vi "Destroy.vi"(8 "error in (no error)":errorcluster caption="错误输入（无错误）", 11 "User Event Collection 输入":refnum<class "User Event Collection.lvclass"> caption="DNL_LabVIEW Object in") -> (0 "error out":errorcluster caption="错误输出", 3 "User Event Collection 输出":refnum<class "User Event Collection.lvclass"> caption="DNL_LabVIEW Object out")   [LabVIEW 2013, in "User Event Collection.lvclass"]
uses:
  User Event Collection.lvclass
  User Event Collection.lvclass/User Event Collection.ctl
  <resource>/importtools/Common/Event/NISAST Event.lvclass
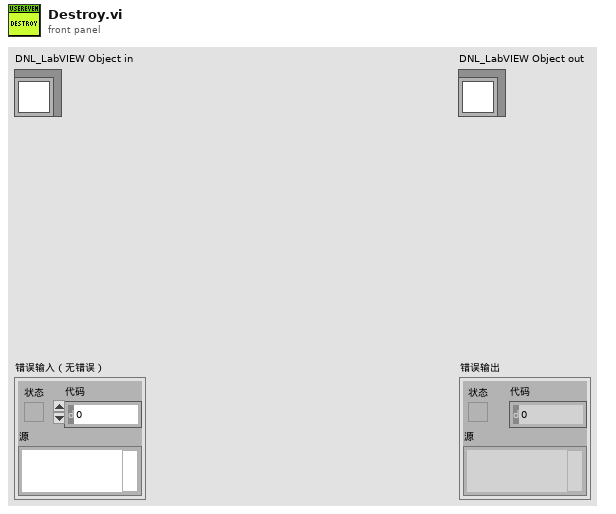
[diagram p1: front panel]
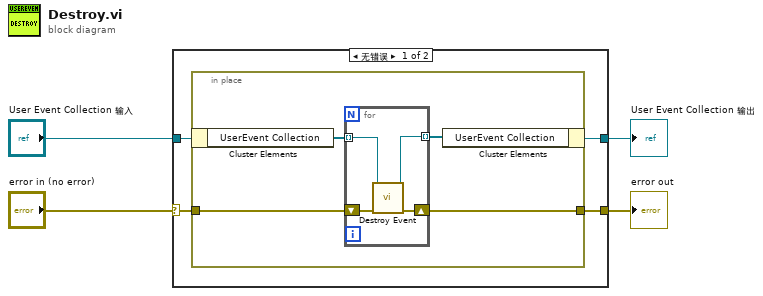
[diagram p0: block diagram]
diagram:
  n1 = case shown="无错误" "error in (no error)" {
    selector: "error in (no error)" -> [w8 w18]
    tunnel: [w7 w18] -> w3
    tunnel: [w5 w17] -> w1
    tunnel: "User Event Collection 输入" -> [w6 w17]
    frame No Error {
      n2 = in-place {
        in-place-border: w8 -> [w12]
        in-place-border: [w11] -> w7
        n3 = in-place-cluster #1(w6) -> ("UserEvent Collection"=w10:refnum<class "NISAST Event.lvclass">[])
        n4 = for {
          shift-right: [w15] -> w11
          shift-left: w12 -> [w16]
          tunnel: w10 -> [w14] mode=indexing
          tunnel: [w13] -> w9 mode=indexing
          n5 = call-dynamic "Destroy Event.vi"("error in (no error)"=w16, "Event in"=w14) -> ("error out"=w15:errorcluster, "Event out"=w13:refnum<class "NISAST Event.lvclass">)  [unwired: 8 in]
        }
        n6 = in-place-cluster #1("UserEvent Collection"=w9) -> (w5:refnum<class "User Event Collection.lvclass">)
      }
    }
    frame Error {
    }
  }
  "error out" <- w3
  "User Event Collection 输出" <- w1
